vi "TCP disconnect.vi"(8 "error in (no error)":errorcluster, 11 "connection ID":refnum<k5>) -> (0 "error out":errorcluster)   [LabVIEW 2019, in "ACSVcontrol-driver.lvlib"]
doc: "Close TCP connection. Connection is closed always, even in the case of error."
uses:
  ACSVcontrol-driver.lvlib
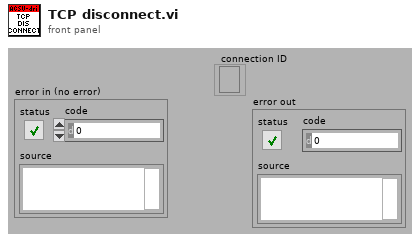
[diagram p1: front panel]
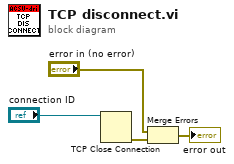
[diagram p0: block diagram]
diagram:
  n1 = TCP Close Connection(connection ID="connection ID") -> (error out=w3:errorcluster)  [unwired: 2 in, 1 out]
  n2 = Merge Errors("error in (no error)", w3) -> (→"error out":errorcluster)
